vi "Stop.vi"(10 "Code":i32, 11 "Test 1 in":refnum<class "Test Caller.lvclass">) -> (3 "Test 1 out":refnum<class "Test Caller.lvclass">)   [LabVIEW 2020, in "Scratchpad.lvlib" / "Test Caller.lvlib" / "Test Caller.lvclass"]
uses:
  Test Caller.lvclass
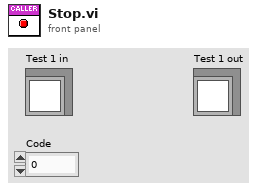
[diagram p1: front panel]
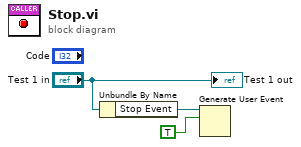
[diagram p0: block diagram]
diagram:
  n1 = Unbundle By Name("Test 1 in") -> ("Stop Event"=w2:refnum<user-event>)
  n2 = Generate User Event(user event=w2, event data cluster=TRUE ("event data")) -> ()  [unwired: 2 in, 2 out]
  "Test 1 out" <- "Test 1 in"
